vi "DefaultFromIni.vi"(8 "error in (no error)":errorcluster, 11 "SiemensDigitalEnergyMeter in":refnum<class "SiemensDigitalEnergyMeter.lvclass">) -> (0 "error out":errorcluster, 3 "SiemensDigitalEnergyMeter out":refnum<class "SiemensDigitalEnergyMeter.lvclass">)   [LabVIEW 2018, in "SensorPlugins.lvlib" / "SiemensDigitalEnergyMeter.lvclass"]
doc: "This VI opens the configuration INI file and loads the information from the file into the class cluster."
uses:
  SiemensDigitalEnergyMeter.lvclass
  C:/Program Files (x86)/National Instruments/LabVIEW 2018/user.lib/NIST/BaseClasses/BasePlugin_class/BasePlugin.lvclass
  TypeDefinitions/SiemensDigitalEnergyMeterControls.ctl
  <userlib>/NIST/BaseClasses/BasePlugin_class/BasePlugin.lvclass/BasePlugin.ctl
  TypeDefinitions/MeasurementControls.ctl
  <userlib>/NIST/BaseClasses/BasePlugin_class/Accessors/Read PluginIniFilePath.vi
  <vilib>/Utility/error.llb/Error Cluster From Error Code.vi
  <vilib>/ErrorRing/Error Ring.xnode
  <vilib>/Utility/config.llb/NI_LVConfig.lvlib
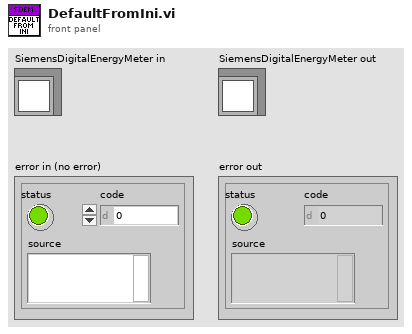
[diagram p1: front panel]
types:
  T1 = typedef "SensorPlugins.lvlib/SiemensDigitalEnergyMeter.lvclass/MeasurementControls.ctl" = cluster{"Measurement RefreshTime (ms)":u32, "Measurement Name":string}
  T2 = typedef "SensorPlugins.lvlib/SiemensDigitalEnergyMeter.lvclass/SiemensDigitalEnergyMeterControls.ctl" = cluster{"Measurement(s)":u16[], "Configuration Commands":string, "Use Measurement Commands Text Box?":bool, "Measurement Commands":string, "Connected?":bool, "Serial Number":string, "IP Address":string, "Port (502)":u16, "Unit ID":u8, "Serial Type":enum16{"RTU", "ASCII"}, "VISA Resource Name":refnum<visa-resource-name>, "Using TCP?":bool}[]
  T3 = typedef "NI_LVConfig.lvlib/Config Data RefNum.ctl" = refnum<k1>
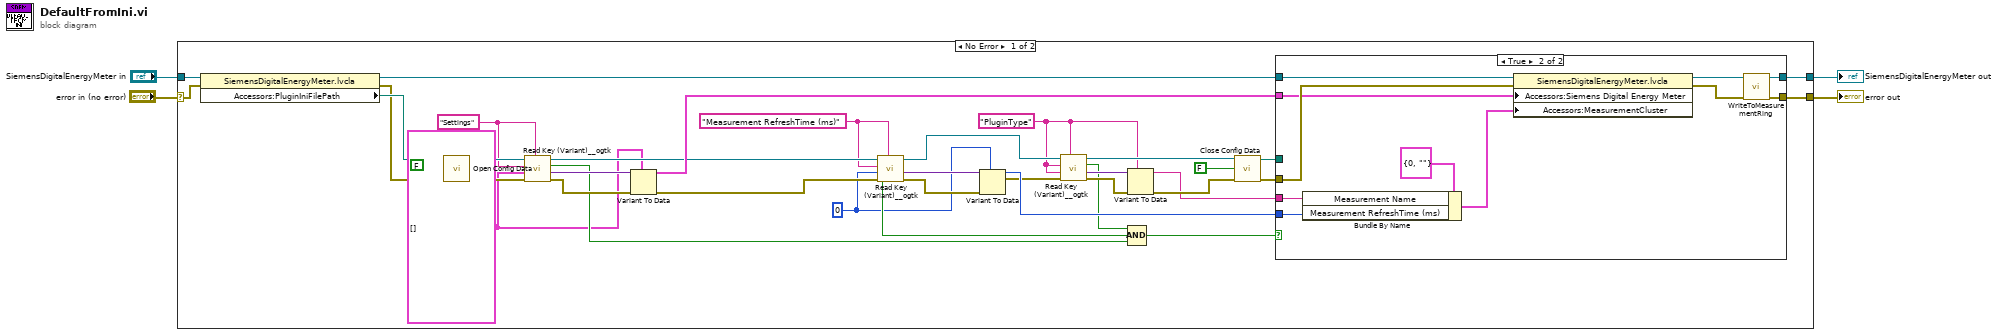
[diagram p0: block diagram]
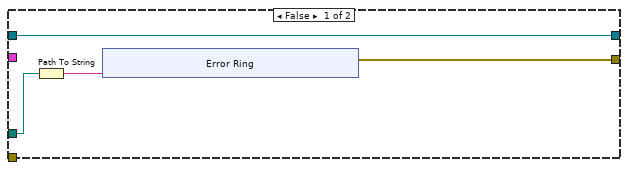
[diagram p2: hidden frame]
diagram:
  n1 = case shown="No Error" "error in (no error)" {
    selector: "error in (no error)" -> [w40 w64]
    tunnel: "SiemensDigitalEnergyMeter in" -> [w41 w65]
    tunnel: [w33 w65] -> w2
    tunnel: [w29 w64] -> w1
    frame No Error {
      w5 = "PluginType" ("section")
      w14 = u32 0 ("Measurement RefreshTime (ms)")
      w15 = T2 [] ("Siemens Digital Energy Meter")
      w17 = "Measurement RefreshTime (ms)" ("section")
      w26 = "Settings" ("section")
      n2 = property class="SiemensDigitalEnergyMeter.lvcla"(reference=w41, error in=w40) -> (reference out=w34:refnum<class "SiemensDigitalEnergyMeter.lvclass">, error out=w37:errorcluster, "Accessors:PluginIniFilePath"=w39:path)
      n3 = call <vilib>:"Open Config Data.vi"("error in (no error)"=w37, "create file if necessary (T)"=FALSE, "configuration file path"=w39) -> ("error out"=w35:errorcluster, "refnum"=w36:T3)  [unwired: 6 in, 1 out]
      n4 = call <userlib>:"Read Key (Variant)__ogtk.vi"("section"=w26, "error in (no error)"=w35, "type"=w15, "key (optional)"=w26, "refnum"=w36) -> ("error out"=w31:errorcluster, "key-value"=w32:variant, "found?"=w24:bool, "refnum out"=w19:T3)  [unwired: 3 in]
      n5 = Variant To Data(error in=w31, type=w15, Variant=w32) -> (data=w30:T2, error out=w20:errorcluster)
      n6 = call <userlib>:"Read Key (Variant)__ogtk.vi"("section"=w17, "error in (no error)"=w20, "type"=w14, "key (optional)"=w17, "refnum"=w19) -> ("error out"=w22:errorcluster, "key-value"=w21:variant, "found?"=w18:bool, "refnum out"=w12:T3)  [unwired: 3 in]
      n7 = Variant To Data(error in=w22, type=w14, Variant=w21) -> (data=w16:u32, error out=w13:errorcluster)
      n8 = call <userlib>:"Read Key (Variant)__ogtk.vi"("section"=w5, "error in (no error)"=w13, "type"=w5, "key (optional)"=w5, "refnum"=w12) -> ("error out"=w10:errorcluster, "key-value"=w8:variant, "found?"=w7:bool, "refnum out"=w11:T3)  [unwired: 3 in]
      n9 = Variant To Data(error in=w10, type=w5, Variant=w8) -> (data=w6:string, error out=w9:errorcluster)
      n10 = Compound Arithmetic op=AND(w7, w18, w24) -> (w25:bool)
      n11 = call <vilib>:"Close Config Data.vi"("error in (no error)"=w9, "write file if changed (T)"=FALSE, "refnum"=w11) -> ("error out"=w28:errorcluster, "file path"=w23:path)  [unwired: 7 in]
      n12 = case shown="True" w25 {
        tunnel: w34 -> [w45 w63]
        tunnel: [w45 w57] -> w33
        tunnel: w30 -> [_ w61]
        tunnel: [w42 w59] -> w29
        tunnel: w28 -> [_ w62]
        tunnel: w23 -> [w43 _]
        tunnel: w16 -> [_ w55]
        tunnel: w6 -> [_ w54]
        frame False {
          n13 = Path To String(path=w43) -> (string=w44:string)
          n14 = xnode "Error Ring"("parameter 0"=w44) -> ("error out"=w42:errorcluster)
        }
        frame True {
          n15 = Bundle By Name(cluster=T1 {"Measurement RefreshTime (ms)"=0, "Measurement Name"=""} ("MeasurementCluster"), "Measurement Name"=w54, "Measurement RefreshTime (ms)"=w55) -> (w53:T1)
          n16 = property class="SiemensDigitalEnergyMeter.lvcla"(reference=w63, error in=w62, "Accessors:Siemens Digital Energy Meter"=w61, "Accessors:MeasurementCluster"=w53) -> (reference out=w58:refnum<class "SiemensDigitalEnergyMeter.lvclass">, error out=w60:errorcluster)
          n17 = call-dynamic "WriteToMeasurementRing.vi"("error in (no error)"=w60, "SiemensDigitalEnergyMeter in"=w58) -> ("error out"=w59:errorcluster, "SiemensDigitalEnergyMeter out"=w57:refnum<class "SiemensDigitalEnergyMeter.lvclass">)  [unwired: 8 in]
        }
      }
    }
    frame Error {
    }
  }
  "error out" <- w1
  "SiemensDigitalEnergyMeter out" <- w2
